vi "PCO_ArmCamera.vi"(8 "error in (no error)":errorcluster {"code" format="%x"}, 11 "ph":u64) -> (0 "error out":errorcluster {"code" format="%x"}, 2 "ErrorMessage":i32 format="%x", 3 "ph out":u64)   [LabVIEW 2019, in "SDK.lvlib" / "GeneralCameraControl.lvlib"]
doc: "<b>Description:</b>\nThis function does arm, this means prepare the camera for a following recording. All configurations and settings made up to this moment are accepted, validated and the internal settings of the camera are prepared. If the arm was successful the camera state is changed to [armed] and the camera is able to start image recording immediately, when Recording State is set to [run].\n\nThe command will be rejected, if Recording State is [run], see PCO_GetRecordingState.\n\nOn power up the camera is in state [not armed] and Recording State [stop].\nCamera arm state is changed to [not armed], when settings are changed, with the following exception. Camera arm state is not changed, when settings related to exposure time will be done during Recording State [run].\n\n<b>Supported camera type:</b>\nAll cameras\n\n<b>Descriptor dependency:</b>\nNone"
uses:
  GeneralCameraControl.lvlib
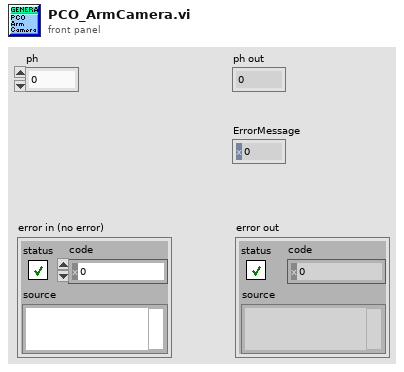
[diagram p1: front panel]
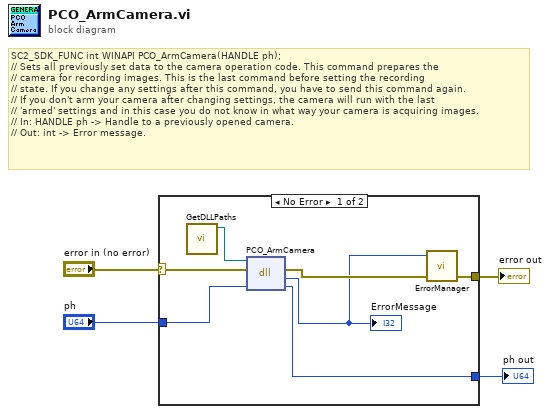
[diagram p0: block diagram]
diagram:
  # "SC2_SDK_FUNC int WINAPI PCO_ArmCamera(HANDLE ph);\n// Sets all previously set data to the camera operation code. This command prepares the\n// camera for recording images. This is the last command before setting the recording\n// state. If you change any settings after this command, you have to send this command again.\n// If you don't arm your camera after changing settings, the camera will run with the last\n// 'armed' settings and in this case you do not know in what way your camera is acquiring images.\n// In: HANDLE ph -> Handle to a previously opened camera.\n// Out: int -> Error message."
  n1 = case shown="No Error" "error in (no error)" {
    selector: "error in (no error)" -> [w7 w13]
    tunnel: [w10 w13] -> w4
    tunnel: [w8 w12] -> w3
    tunnel: "ph" -> [w6 w12]
    frame No Error {
      n2 = call "GetDLLPaths.vi"() -> ("SC2_Cam_Path"=w5:path)  [unwired: 9 in, 2 out]
      n3 = dll-call lib="?" fn="PCO_ArmCamera"(path in=w5, error in=w7, "ph"=w6) -> (error out=w11:errorcluster, "return type"=w9:i32, "ph"=w8:u64)  [unwired: 1 in, 1 out]
      "ErrorMessage" <- w9
      n4 = call "ErrorManager.vi"("error in (no error)"=w11, "error code"=w9) -> ("error out"=w10:errorcluster)  [unwired: 3 in]
    }
    frame Error {
    }
  }
  "error out" <- w4
  "ph out" <- w3
